vi "Station_Port_Dialog_USB.vi"(5 "Enable":bool=TRUE, 7 "Error in":errorcluster, 8 "Station ID in":i32 min=0, 9 "Baud rate in":i32(ring)=19200 items=["1200"=1200, "2400"=2400, "4800"=4800, "9600"=9600, "14400"=14400, "19200"=19200], 10 "COM port in":i32 min=0) -> (0 "Error out":errorcluster, 1 "Station ID out":i32, 2 "Baud rate out":i32, 3 "COM port out":i32, 4 "OK":bool, 6 "Help?":bool)   [LabVIEW 2013]
doc: "Displays a standard dialog box that prompts users to enter information, such as a user name and password.\n--------------------\n\nThis Express VI is configured as follows:\n\nMessage to Display to the User:There is a problem in communication with the Vantage Pro console. Check if the console is properly connected with your PC and that you selected the correct COM port number (you can find this number at 'device manager' (apparaatbeheer)).\n\nMoreover select the correct baud rate (19200).\n\nFinally, select the HiSPARC Station ID in (you can find your ID in the file 'Z:\\persistent\\config.ini').\nThe inputs are: \nNumber: COM Poort\nNumber: Baud rate\nNumber: Station ID"
panel:
  out "String":string="Please select to connect:\n\n- Station ID\n  - Identifier for your station distributed together with your certificate\n    (required during software installation)\n  - Usually the same ID as your cosmic ray detector\n  - The ID of your cosmic ray station is stored in: \\persistent\\config.ini"
  in  "Station ID":i32 min=0
  in  "OK":bool
  in  "Stop?":bool
  in  "Help?":bool
  in  "OK1":bool
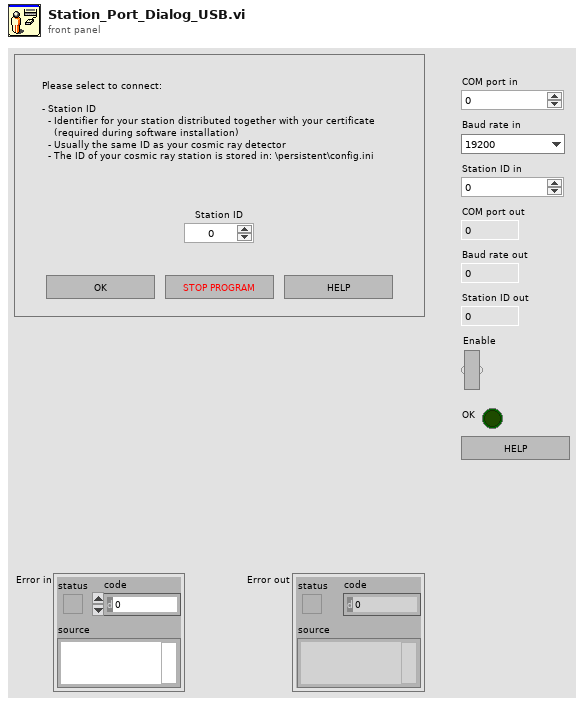
[diagram p1: front panel]
types:
  T1 = cluster{"Input Name":string, "Input Data Type":i32}[]
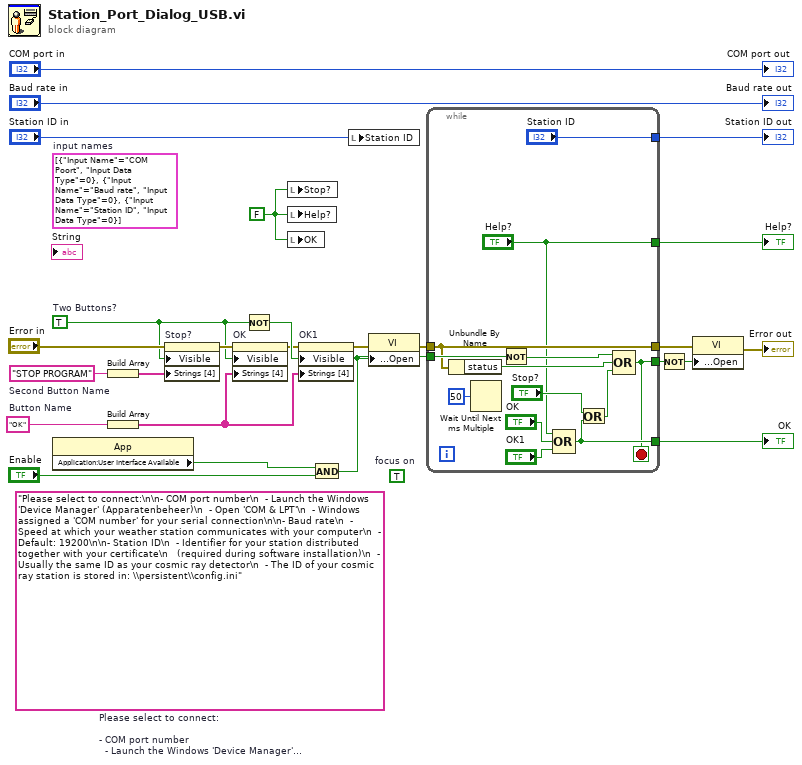
[diagram p0: block diagram]
diagram:
  w3 = FALSE ("Help?")
  (unwired) "Please select to connect:\n\n- COM port number\n  - Launch the Windows 'Device Manager' (Apparatenbeheer)\n  - Open 'COM & LPT'\n  - Windows assigned a 'COM number' for your serial connection\n\n- Baud rate\n  - Speed at which your weather station communicates with your computer\n  - Default: 19200\n\n- Station ID\n  - Identifier for your station distributed together with your certificate\n   (required during software installation)\n  - Usually the same ID as your cosmic ray detector\n  - The ID of your cosmic ray station is stored in: \\persistent\\config.ini"  # Please select to connect:  - COM port number   - Launch the Windows 'Device Manager' (Apparatenbeheer)   - Open 'COM & LPT'   - Windows assigned a 'COM number' for your serial connection  - Baud rate   - Speed at which your weather station communicates with your computer   - Default: 19200  - Station ID   - Identifier for your station distributed together with your certificate    (required during software installation)   - Usually the same ID as your cosmic ray detector   - The ID of your cosmic ray station is stored in: \persistent\config.ini
  (unwired) TRUE  # focus on
  (unwired) T1 [{"Input Name"="COM Poort", "Input Data Type"=0}, {"Input Name"="Baud rate", "Input Data Type"=0}, {"Input Name"="Station ID", "Input Data Type"=0}]  # input names
  w21 = "STOP PROGRAM"  # Second Button Name
  w20 = "OK"  # Button Name
  w7 = TRUE  # Two Buttons?
  n1 = property class="App"() -> ("Application:User Interface Available"=w12:bool)  [unwired: 2 in, 2 out]
  n2 = Build Array(w21) -> (w9:string[])
  n3 = Build Array(w20) -> (w5:string[])
  n4 = property on="Stop?" class="Bool (strict)"(error in="Error in", "Visible"=w7, "Strings [4]"=w9) -> (error out=w8:errorcluster)  [unwired: 1 in, 1 out]
  n5 = property on="OK" class="Bool (strict)"(error in=w8, "Visible"=w7, "Strings [4]"=w5) -> (error out=w6:errorcluster)  [unwired: 1 in, 1 out]
  n6 = Not(x=w7) -> (.not. x?=w24:bool)
  n7 = local write "Stop?"(w3) -> ()
  n8 = local write "Help?"(w3) -> ()
  n9 = local write "OK"(w3) -> ()
  n10 = property on="OK1" class="Bool"(error in=w6, "Visible"=w24, "Strings [4]"=w5) -> (error out=w19:errorcluster)  [unwired: 1 in, 1 out]
  n11 = And(x=w12, y="Enable") -> (x .and. y?=w15:bool)
  n12 = local write "Station ID"("Station ID in") -> ()
  n13 = property class="VI"(error in=w19, "Front Panel Window:Open"=w15) -> (error out=w18:errorcluster)  [unwired: 1 in, 1 out]
  n14 = while "Main While Loop" {
    tunnel: [w37] -> w25
    tunnel: w15 -> [w36]
    tunnel: [w34] -> w22
    tunnel: w18 -> [w33]
    tunnel: [w33] -> w17
    tunnel: ["Station ID"] -> w14
    tunnel: ["Help?"] -> w4
    stop <- w34 stop-if-true
    n15 = Unbundle By Name(w33) -> ("status"=w31:bool)
    n16 = Wait Until Next ms Multiple(millisecond multiple=u32 50) -> ()  [unwired: 1 out]
    n17 = Not(x=w36) -> (.not. x?=w35:bool)
    n18 = Compound Arithmetic op=OR("Help?", "OK", "OK1") -> (w37:bool)
    n19 = Or(x="Stop?", y=w37) -> (x .or. y?=w32:bool)
    n20 = Compound Arithmetic op=OR(w35, w31, w32) -> (w34:bool)
  }
  "OK" <- w25
  "Station ID out" <- w14
  "Help?" <- w4
  n21 = Not(x=w22) -> (.not. x?=w23:bool)
  n22 = property class="VI"(error in=w17, "Front Panel Window:Open"=w23) -> (error out=→"Error out":errorcluster)  [unwired: 1 in, 1 out]
  "COM port out" <- "COM port in"
  "Baud rate out" <- "Baud rate in"
